vi "CreateLinPosStrings.vi"(8 "error in (no error)":errorcluster, 9 "Z/F(x) val":dbl, 10 "Coord":cluster{"X":dbl, "Y":dbl}, 11 "IntensityGraph in":refnum<vi>) -> (0 "error out":errorcluster, 2 "Lin String out":string, 3 "Pos String out":string)   [LabVIEW 2023]
doc: "Produce a new Lin and Pos strings from a single point data"
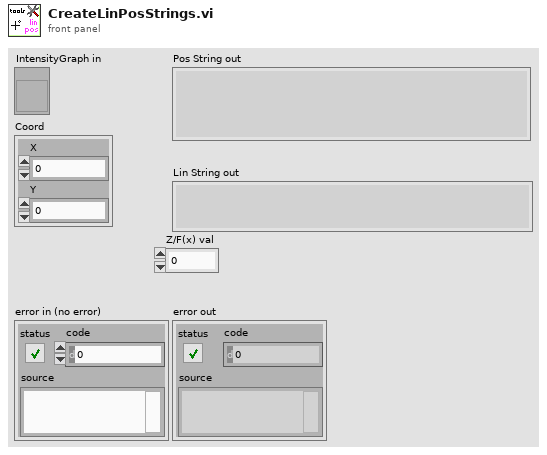
[diagram p1: front panel]
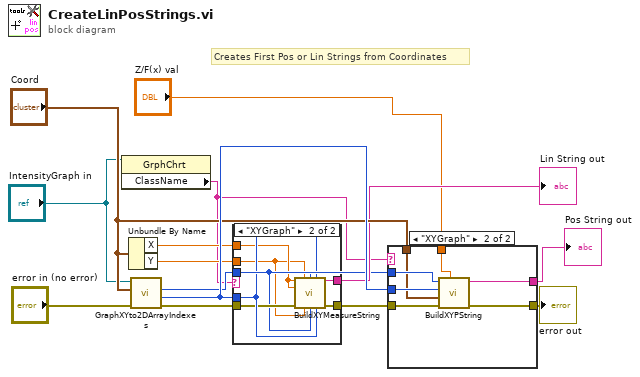
[diagram p0: block diagram]
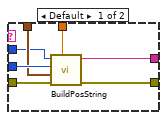
[diagram p2: hidden frame]
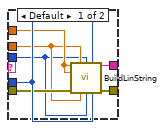
[diagram p3: hidden frame]
diagram:
  # "Creates First Pos or Lin Strings from Coordinates"
  n1 = property class="GrphChrt"(reference="IntensityGraph in") -> ("ClassName"=w2:string)  [unwired: 1 in, 2 out]
  n2 = Unbundle By Name("Coord") -> ("X"=w6:dbl, "Y"=w5:dbl)
  n3 = call "GraphXYto2DArrayIndexes.vi"("error in (no error)"="error in (no error)", "XY"="Coord", "IntensityGraph in"="IntensityGraph in") -> ("error out"=w7:errorcluster, "Y Index"=w12:i32, "X Index"=w4:i32)  [unwired: 5 in, 1 out]
  n4 = case shown="\"XYGraph\"" w2 {
    tunnel: [w21 w28] -> w13
    tunnel: w12 -> [w20 w27]
    tunnel: [w19 w26] -> w9
    tunnel: w7 -> [w18 w25]
    tunnel: w6 -> [w17 w24]
    tunnel: w5 -> [w16 w23]
    tunnel: w4 -> [w15 w22]
    frame Default {
      n5 = call "BuildLinString.vi"("X0"=w17, "Y0"=w16, "X0 graph pixels"=w15, "Y0 graph pixels"=w20, "X1"=w17, "error in (no error)"=w18, "Y1"=w16, "X1 graph pixels"=w15, "Y1 graph pixels"=w20) -> ("String"=w19:string, "error out"=w21:errorcluster)  [unwired: 5 in]
    }
    frame "XYGraph" {
      n6 = call "BuildXYMeasureString.vi"("X0"=w24, "Y0"=w23, "X0 graph pixels"=w22, "Y0 graph pixels"=w27, "X1"=w24, "error in (no error)"=w25, "Y1"=w23, "X1 graph pixels"=w22, "Y1 graph pixels"=w27) -> ("String"=w26:string, "error out"=w28:errorcluster)  [unwired: 5 in]
    }
  }
  "Lin String out" <- w9
  n7 = case shown="\"XYGraph\"" w2 {
    tunnel: [w35 w38] -> w14
    tunnel: w13 -> [w34 w39]
    tunnel: w12 -> [w33 w41]
    tunnel: "Z/F(x) val" -> [w32 w36]
    tunnel: [w31 w37] -> w11
    tunnel: "Coord" -> [w30 w40]
    tunnel: w4 -> [w29 w42]
    frame Default {
      n8 = call "BuildPosString.vi"("Z val"=w32, "error in (no error)"=w34, "XY"=w30, "Y graph pixels"=w33, "X graph pixels"=w29) -> ("error out"=w35:errorcluster, "String"=w31:string)  [unwired: 5 in]
    }
    frame "XYGraph" {
      n9 = call "BuildXYPString.vi"("Z val"=w36, "error in (no error)"=w39, "XY"=w40, "Y graph pixels"=w41, "X graph pixels"=w42) -> ("error out"=w38:errorcluster, "String"=w37:string)  [unwired: 5 in]
    }
  }
  "error out" <- w14
  "Pos String out" <- w11
